vi "Console Send Error.vi"(0 "error in (no error)":errorcluster) -> (15 "no error":errorcluster)   [LabVIEW 2026, in "MrcLib.lvlib"]
doc: "Appends the LabVIEW error information to the console and DS log."
uses:
  MrcLib.lvlib
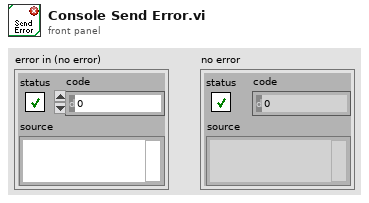
[diagram p1: front panel]
types:
  T1 = typedef "MRC String.ctl" = cluster{"pointer":u64, "length":u64}
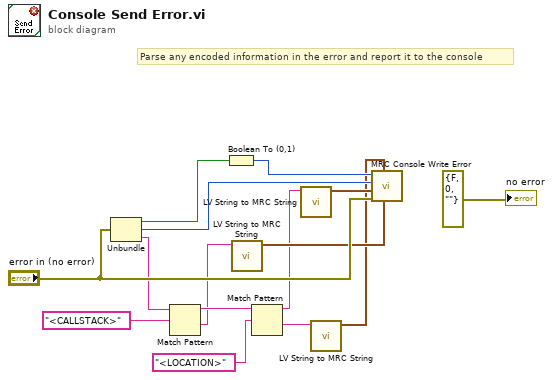
[diagram p0: block diagram]
diagram:
  # "Parse any encoded information in the error and report it to the console"
  n1 = Unbundle("error in (no error)") -> ("status"=w14:bool, "code"=w12:i32, "source"=w8:string)
  n2 = Match Pattern(string=w8, regular expression="<CALLSTACK>" ("string")) -> (before substring=w7:string, after substring=w6:string)  [unwired: 1 in, 2 out]
  n3 = Boolean To (0,1)(Boolean=w14) -> (0, 1=w13:i16)
  n4 = call "LV String to MRC String.vi"("LV String"=w6) -> ("MRC String"=w5:T1)  [unwired: 10 in]
  n5 = Match Pattern(string=w7, regular expression="<LOCATION>" ("string")) -> (before substring=w2:string, after substring=w3:string)  [unwired: 1 in, 2 out]
  n6 = call "LV String to MRC String.vi"("LV String"=w2) -> ("MRC String"=w11:T1)  [unwired: 10 in]
  n7 = call "LV String to MRC String.vi"("LV String"=w3) -> ("MRC String"=w4:T1)  [unwired: 10 in]
  n8 = call "MRC Console Write Error.vi"("stackTrace"=w5, "location"=w4, "error in (no error)"="error in (no error)", "message"=w11, "errorCode"=w12, "isError"=w13) -> ()  [unwired: 5 in, 1 out]
  "no error" <- errorcluster {"status"=FALSE, "code"=0, "source"=""} ("error out")
